vi "Send Command String.vi"(8 "error in (no error)":errorcluster, 10 "Command String":string, 11 "NMR in":refnum<class "NMR.lvclass">) -> (0 "error out":errorcluster, 3 "NMR out":refnum<class "NMR.lvclass">)   [LabVIEW 2011, in "NMR.lvclass"]
uses:
  NMR.lvclass
  NMR.lvclass/NMR.ctl
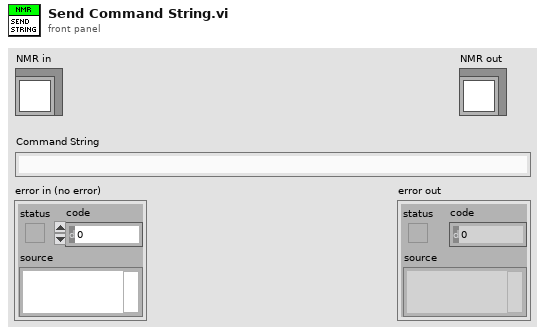
[diagram p1: front panel]
types:
  T1 = typedef "NMR.lvclass/Communication Channel.ctl" = enum16{"VISA", "DLL"}
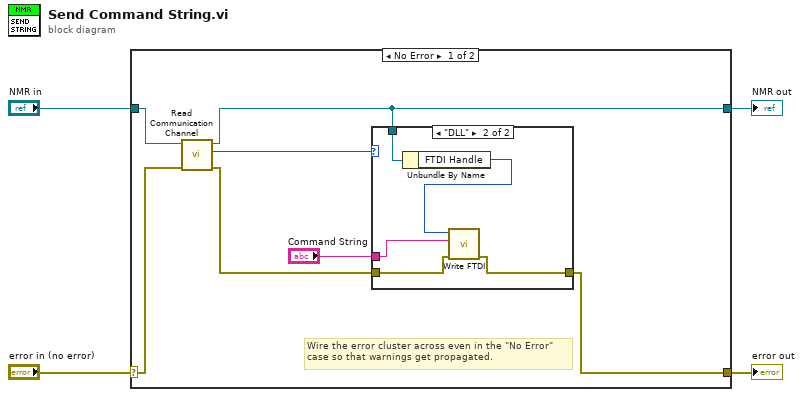
[diagram p0: block diagram]
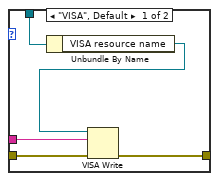
[diagram p2: hidden frame]
diagram:
  n1 = case shown="No Error" "error in (no error)" {
    selector: "error in (no error)" -> [w10 w23]
    tunnel: [w7 w23] -> w3
    tunnel: [w5 w22] -> w1
    tunnel: "NMR in" -> [w11 w22]
    frame No Error {
      # "Wire the error cluster across even in the \"No Error\"\ncase so that warnings get propagated."
      n2 = call-dynamic "Read Communication Channel.vi"("error in (no error)"=w10, "NMR in"=w11) -> ("error out"=w8:errorcluster, "Communication Channel"=w9:T1, "NMR out"=w5:refnum<class "NMR.lvclass">)  [unwired: 7 in]
      n3 = case shown="\"DLL\"" w9 {
        tunnel: w8 -> [w16 w18]
        tunnel: [w15 w17] -> w7
        tunnel: "Command String" -> [w14 w19]
        tunnel: w5 -> [w13 w21]
        frame "VISA", Default {
          n4 = Unbundle By Name(w13) -> ("VISA resource name"=w12:refnum<visa-resource-name>)
          n5 = VISA Write(VISA resource name=w12, write buffer=w14, error in (no error)=w16) -> (error out=w15:errorcluster)  [unwired: 2 out]
        }
        frame "DLL" {
          n6 = Unbundle By Name(w21) -> ("FTDI Handle"=w20:u32)
          n7 = call "Write FTDI.vi"("error in (no error)"=w18, "Write STR"=w19, "FTDI Handle In"=w20) -> ("error out"=w17:errorcluster)  [unwired: 6 in, 2 out]
        }
      }
    }
    frame Error {
    }
  }
  "error out" <- w3
  "NMR out" <- w1
